vi "Do.vi"(8 "error in (no error)":errorcluster, 10 "Actor in":refnum<class "Actor.lvclass">, 11 "StartTask Msg":refnum<class "StartTask Msg.lvclass">) -> (0 "error out":errorcluster, 2 "Actor out":refnum<class "Actor.lvclass">)   [LabVIEW 2025, in "DAQ_Module.lvlib" / "StartTask Msg.lvclass"]
doc: "This VI delivers the message to the actor by calling the appropriate method(s) on the actor."
uses:
  StartTask Msg.lvclass
  <vilib>/ActorFramework/Actor/Actor.lvclass
  StartTask Msg.lvclass/StartTask Msg.ctl
  DAQ_Module/DAQ_Module.lvclass
  9ef47adc-f318-494c-9b8b-6df3216d6863.vi
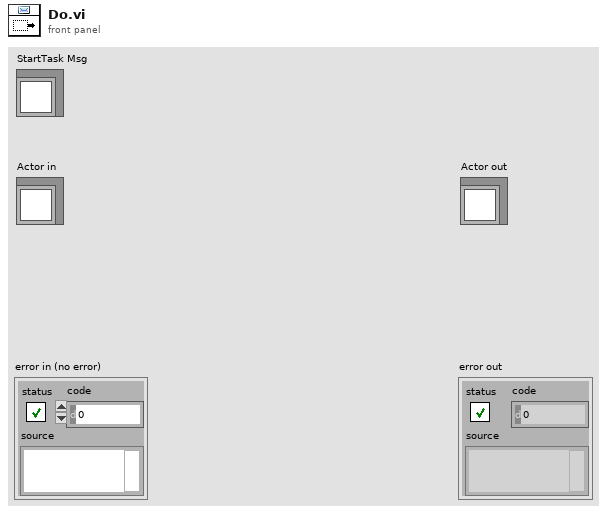
[diagram p1: front panel]
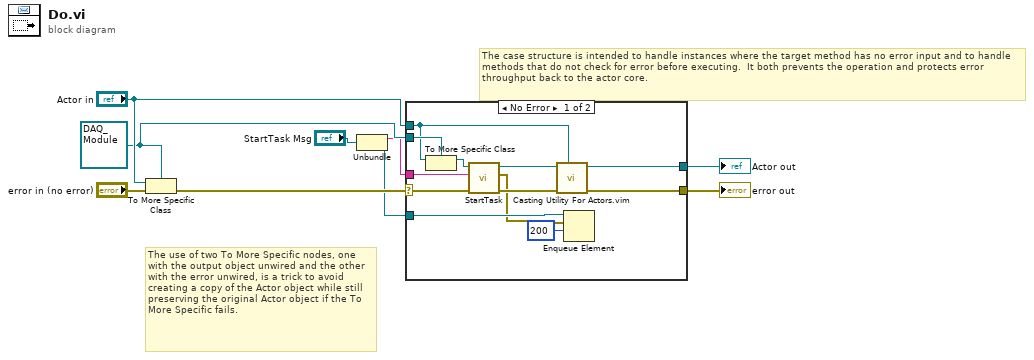
[diagram p0: block diagram]
diagram:
  w3 = refnum<class "DAQ_Module.lvclass"> refnum ("Actor in")
  # "The use of two To More Specific nodes, one with the output object unwired and the other with the error unwired, is a trick to avoid creating a copy of the Actor object while still preserving the original Actor object if the To More Specific fails."
  # "The case structure is intended to handle instances where the target method has no error input and to handle methods that do not check for error before executing.  It both prevents the operation and protects error throughput back to the actor core."
  n1 = To More Specific Class(target class=w3, reference="Actor in", error in="error in (no error)") -> (error out=w7:errorcluster)  [unwired: 1 out]
  n2 = Unbundle("StartTask Msg") -> (w2:string, w1:refnum<queue>)
  n3 = case shown="No Error" w7 {
    selector: w7 -> [w21 w23]
    tunnel: [w15 w23] -> w6
    tunnel: [w16 w22] -> w5
    tunnel: "Actor in" -> [w18 w22]
    tunnel: w3 -> [w19 _]
    tunnel: w2 -> [w13 _]
    tunnel: w1 -> [w12 _]
    frame No Error {
      n4 = To More Specific Class(target class=w19, reference=w18) -> (specific class reference=w20:refnum<class "DAQ_Module.lvclass">)  [unwired: 1 in, 1 out]
      n5 = call "StartTask.vi"("error in (no error)"=w21, "Task"=w13, "DAQ_Module in"=w20) -> ("error out"=w14:errorcluster, "daq error"=w11:errorcluster, "DAQ_Module out"=w17:refnum<class "DAQ_Module.lvclass">)  [unwired: 6 in]
      n6 = call "Casting Utility For Actors.vim"("type"=w18, "error in (no error)"=w14, "Actor in"=w17) -> ("error out"=w15:errorcluster, "Actor out"=w16:refnum<class "Actor.lvclass">)  [unwired: 7 in]
      n7 = Enqueue Element(queue=w12, element=w11, timeout in ms (-1)=200) -> ()  [unwired: 1 in, 3 out]
    }
    frame Error {
      # "If type check fails, pass the original object out again."
    }
  }
  "error out" <- w6
  "Actor out" <- w5
